vi "zeroing_computations.vi"(0 "done_zeroing":bool, 1 "forces_offset in":dbl[](array[numeric]), 2 "zero_index in":i32, 3 "angle_offset in":dbl, 4 "zero_array":dbl[][](array[numeric]), 5 "zero_angle in":bool, 6 "eld_offset in":dbl[](array[numeric]), 8 "zero_forces in":bool, 9 "zero_eld in":bool, 10 "Boolean 4":bool, 11 "aux_press_offset in":dbl, 12 "Boolean 2":bool, 13 "pitot_press_offset in":dbl, 14 "Boolean 5":bool, 15 "zero_airspeed in":bool, 16 "Boolean 3":bool, 18 "Boolean":bool) -> (17 "pitot_press_offset out":dbl, 19 "aux_press_offset out":dbl, 20 "zero_forces out":bool, 21 "forces_offset out":dbl[](array[numeric]), 22 "angle_offset out":dbl, 23 "zero_angle out":bool, 24 "zero_index out":i32, 25 "eld_offset out":dbl[](array[numeric]), 26 "zero_eld out":bool, 27 "zero_airspeed out":bool)   [LabVIEW 2019]
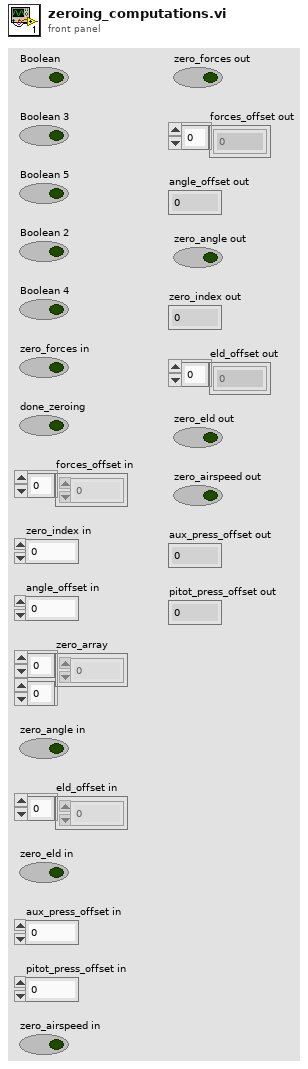
[diagram p1: front panel]
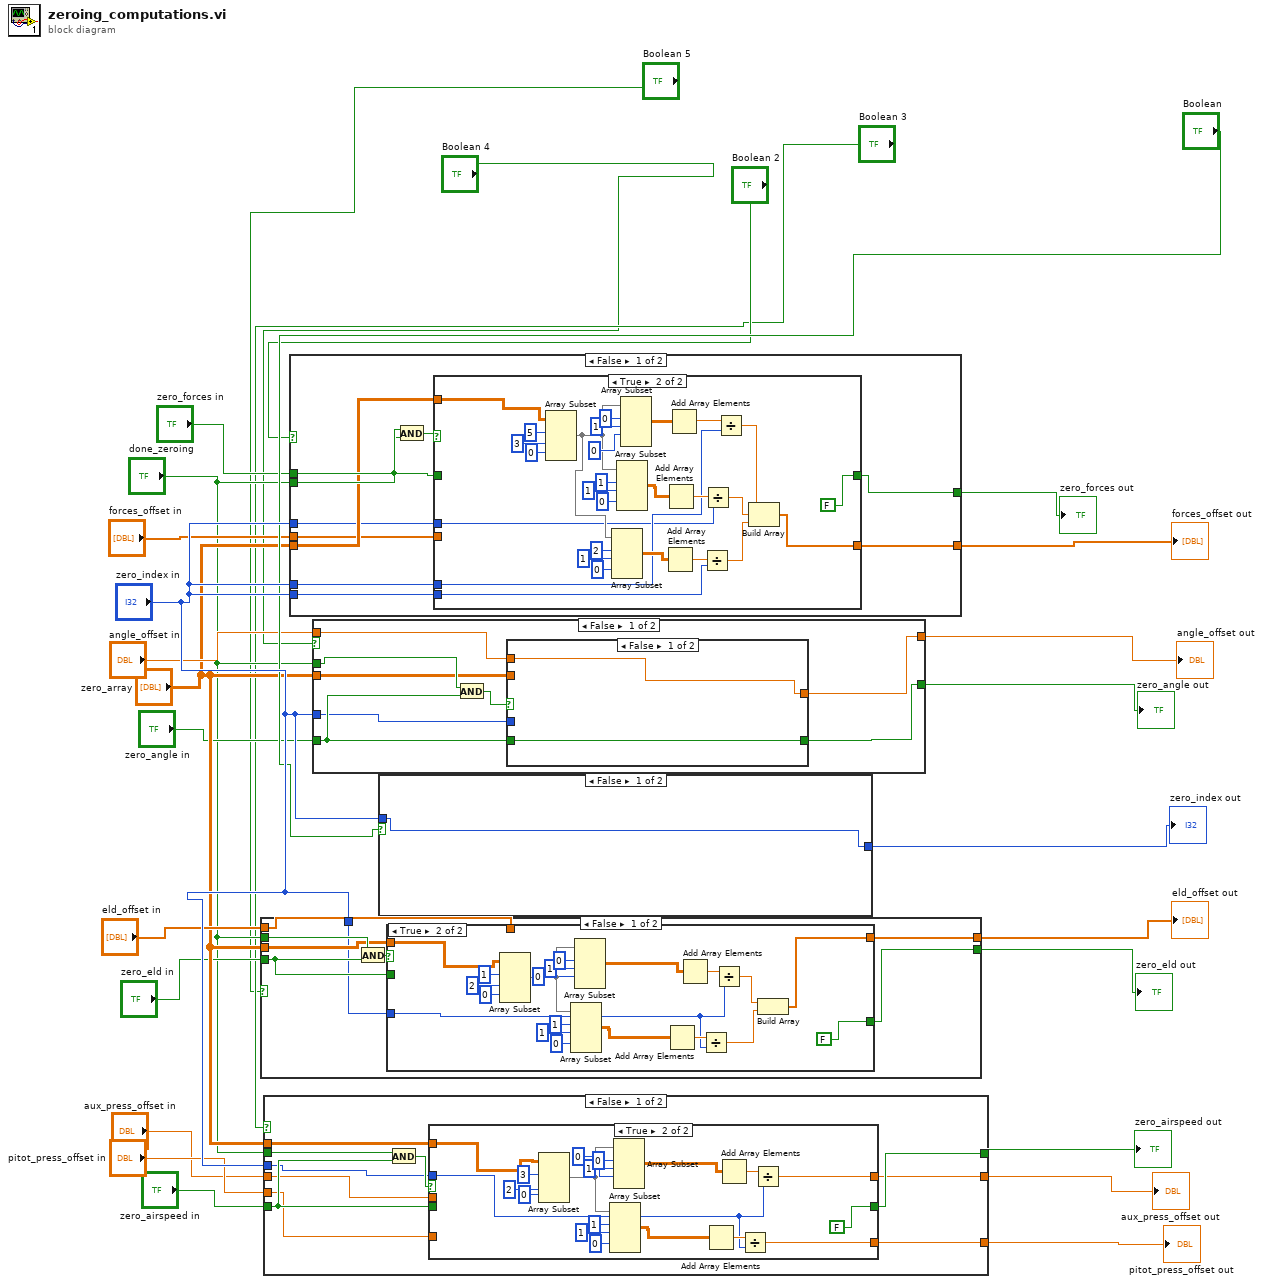
[diagram p0: block diagram]
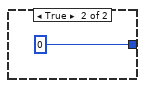
[diagram p2: hidden frame]
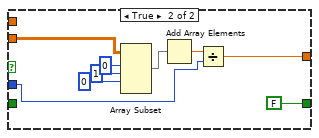
[diagram p9: hidden frame]
diagram:
  n1 = case shown="False" "Boolean 5" {
    selector: "Boolean 5" -> [_ w59]
    tunnel: "done_zeroing" -> [w34 _]
    tunnel: [w33 w59] -> w9
    tunnel: "zero_eld in" -> [w32 _]
    tunnel: "zero_array" -> [w31 _]
    tunnel: [w30 w58] -> w18
    tunnel: "eld_offset in" -> [w29 w58]
    tunnel: "zero_index in" -> [w28 _]
    frame False {
      n2 = And(x=w34, y=w32) -> (x .and. y?=w35:bool)
      n3 = case shown="True" w35 {
        tunnel: [w37 FALSE ("zero_eld")] -> w33
        tunnel: w32 -> [w37 _]
        tunnel: w31 -> [_ w40]
        tunnel: [w36 w39] -> w30
        tunnel: w29 -> [w36 _]
        tunnel: w28 -> [_ w38]
        frame False {
        }
        frame True {
          n4 = Array Subset(array=w40, index (row)=1 ("index"), length (row)=2 ("length"), index (col)=0 ("index")) -> (w49:dbl[][])  [unwired: 1 in]
          n5 = Array Subset(array=w49, index (row)=1 ("index"), length (row)=1 ("length"), index (col)=0 ("index")) -> (w44:dbl[][])  [unwired: 1 in]
          n6 = Array Subset(array=w49, index (row)=0 ("index"), length (row)=1 ("length"), index (col)=0 ("index")) -> (w50:dbl[][])  [unwired: 1 in]
          n7 = Add Array Elements(numeric array=w44) -> (sum=w45:dbl)
          n8 = Add Array Elements(numeric array=w50) -> (sum=w54:dbl)
          n9 = Divide(x=w45, y=w38) -> (x/y=w42:dbl)
          n10 = Divide(x=w54, y=w38) -> (x/y=w43:dbl)
          n11 = Build Array(w43, w42) -> (w39:dbl[])
        }
      }
    }
    frame True {
    }
  }
  "eld_offset out" <- w18
  "zero_eld out" <- w9
  n12 = case shown="False" "Boolean 3" {
    selector: "Boolean 3" -> [_ w94]
    tunnel: "done_zeroing" -> [w68 _]
    tunnel: [w67 w94] -> w10
    tunnel: "zero_airspeed in" -> [w66 _]
    tunnel: "zero_array" -> [w65 _]
    tunnel: [w64 w93] -> w20
    tunnel: [w63 w92] -> w21
    tunnel: "aux_press_offset in" -> [w62 w93]
    tunnel: "pitot_press_offset in" -> [w61 w92]
    tunnel: "zero_index in" -> [w60 _]
    frame False {
      n13 = And(x=w68, y=w66) -> (x .and. y?=w69:bool)
      n14 = case shown="True" w69 {
        tunnel: [w72 FALSE] -> w67
        tunnel: w66 -> [w72 _]
        tunnel: w65 -> [_ w76]
        tunnel: [w71 w75] -> w64
        tunnel: [w70 w74] -> w63
        tunnel: w62 -> [w71 _]
        tunnel: w61 -> [w70 _]
        tunnel: w60 -> [_ w73]
        frame False {
        }
        frame True {
          n15 = Array Subset(array=w76, index (row)=3 ("index"), length (row)=2 ("length"), index (col)=0 ("index")) -> (w83:dbl[][])  [unwired: 1 in]
          n16 = Array Subset(array=w83, index (row)=1 ("index"), length (row)=1 ("length"), index (col)=0 ("index")) -> (w78:dbl[][])  [unwired: 1 in]
          n17 = Array Subset(array=w83, index (row)=0 ("index"), length (row)=1 ("length"), index (col)=0 ("index")) -> (w84:dbl[][])  [unwired: 1 in]
          n18 = Add Array Elements(numeric array=w78) -> (sum=w79:dbl)
          n19 = Add Array Elements(numeric array=w84) -> (sum=w88:dbl)
          n20 = Divide(x=w79, y=w73) -> (x/y=w74:dbl)
          n21 = Divide(x=w88, y=w73) -> (x/y=w75:dbl)
        }
      }
    }
    frame True {
    }
  }
  "pitot_press_offset out" <- w21
  "aux_press_offset out" <- w20
  "zero_airspeed out" <- w10
  n22 = case shown="False" "Boolean 2" {
    selector: "Boolean 2" -> [_ w135]
    tunnel: "done_zeroing" -> [w103 _]
    tunnel: "zero_forces in" -> [w102 _]
    tunnel: "zero_array" -> [w101 _]
    tunnel: [w100 w136] -> w14
    tunnel: "forces_offset in" -> [w99 w136]
    tunnel: "zero_index in" -> [w98 _]
    tunnel: "zero_index in" -> [w97 _]
    tunnel: "zero_index in" -> [w96 _]
    tunnel: [w95 w135] -> w27
    frame False {
      n23 = And(x=w103, y=w102) -> (x .and. y?=w104:bool)
      n24 = case shown="True" w104 {
        tunnel: [w106 FALSE] -> w95
        tunnel: w102 -> [w106 _]
        tunnel: w101 -> [_ w111]
        tunnel: [w105 w110] -> w100
        tunnel: w99 -> [w105 _]
        tunnel: w98 -> [_ w109]
        tunnel: w97 -> [_ w108]
        tunnel: w96 -> [_ w107]
        frame False {
        }
        frame True {
          n25 = Array Subset(array=w111, index (row)=5 ("index"), length (row)=3 ("length"), index (col)=0 ("index")) -> (w118:dbl[][])  [unwired: 1 in]
          n26 = Array Subset(array=w118, index (row)=2 ("index"), length (row)=1 ("length"), index (col)=0 ("index")) -> (w112:dbl[][])  [unwired: 1 in]
          n27 = Array Subset(array=w118, index (row)=1 ("index"), length (row)=1 ("length"), index (col)=0 ("index")) -> (w123:dbl[][])  [unwired: 1 in]
          n28 = Array Subset(array=w118, index (row)=0 ("index"), length (row)=1 ("length"), index (col)=0 ("index")) -> (w128:dbl[][])  [unwired: 1 in]
          n29 = Add Array Elements(numeric array=w112) -> (sum=w114:dbl)
          n30 = Add Array Elements(numeric array=w123) -> (sum=w124:dbl)
          n31 = Add Array Elements(numeric array=w128) -> (sum=w116:dbl)
          n32 = Divide(x=w114, y=w109) -> (x/y=w113:dbl)
          n33 = Divide(x=w124, y=w107) -> (x/y=w117:dbl)
          n34 = Divide(x=w116, y=w108) -> (x/y=w115:dbl)
          n35 = Build Array(w115, w117, w113) -> (w110:dbl[])
        }
      }
    }
    frame True {
    }
  }
  "zero_forces out" <- w27
  "forces_offset out" <- w14
  n36 = case shown="False" "Boolean 4" {
    selector: "Boolean 4" -> [_ w157]
    tunnel: "done_zeroing" -> [w143 _]
    tunnel: "zero_angle in" -> [w142 _]
    tunnel: [w141 w157] -> w8
    tunnel: "zero_array" -> [w140 _]
    tunnel: [w139 w156] -> w16
    tunnel: "angle_offset in" -> [w138 w156]
    tunnel: "zero_index in" -> [w137 _]
    frame False {
      n37 = And(x=w143, y=w142) -> (x .and. y?=w144:bool)
      n38 = case shown="False" w144 {
        tunnel: [w146 FALSE] -> w141
        tunnel: w142 -> [w146 _]
        tunnel: w140 -> [_ w149]
        tunnel: [w145 w148] -> w139
        tunnel: w138 -> [w145 _]
        tunnel: w137 -> [_ w147]
        frame False {
        }
        frame True {
          n39 = Array Subset(array=w149, index (row)=0 ("index"), length (row)=1 ("length"), index (col)=0 ("index")) -> (w151:dbl[][])  [unwired: 1 in]
          n40 = Add Array Elements(numeric array=w151) -> (sum=w152:dbl)
          n41 = Divide(x=w152, y=w147) -> (x/y=w148:dbl)
        }
      }
    }
    frame True {
    }
  }
  "angle_offset out" <- w16
  "zero_angle out" <- w8
  n42 = case shown="False" "Boolean" {
    tunnel: [w158 0] -> w25
    tunnel: "zero_index in" -> [w158 _]
    frame False {
    }
    frame True {
    }
  }
  "zero_index out" <- w25
